vi "Counter.vi"() -> ()   [LabVIEW 2012]
uses:
  <vilib>/DAQmx/read.llb/DAQmx Read (Counter U32 1Chan 1Samp).vi
  <vilib>/DAQmx/create/channels.llb/DAQmx Create Channel (CI-Count Edges).vi
  <vilib>/DAQmx/miscellaneous.llb/DAQmx Fill In Error Info.vi
panel:
  in  "initial count":u32
  out "Det1":u32
  out "Det2":u32
  out "Det3":u32
  out "PSU":u32
  out "error out":errorcluster
  in  "PSU":tag="Dev4/ctr1"
  in  "Det3":tag="Dev4/ctr0"
  in  "Det2":tag="Dev5/ctr1"
  in  "Det1":tag="Dev5/ctr0"
  in  "stop":bool
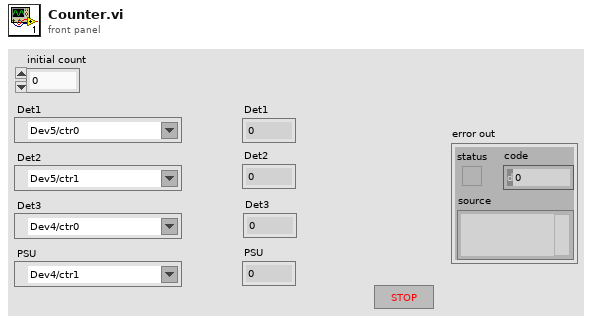
[diagram p1: front panel]
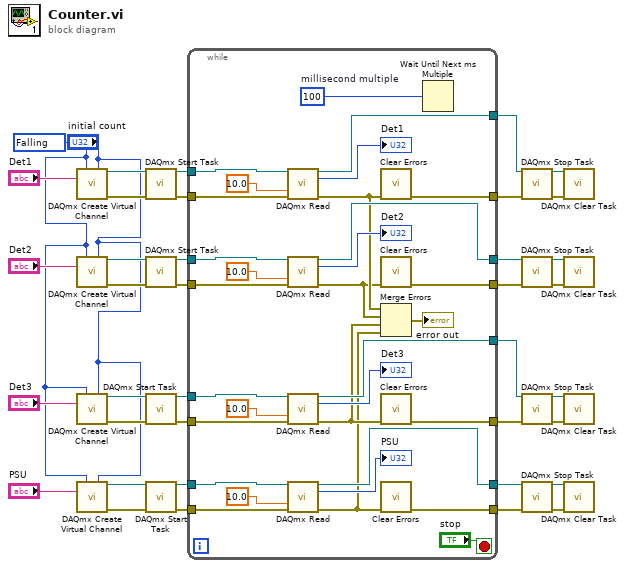
[diagram p0: block diagram]
diagram:
  w1 = 10171 items=["Rising"=10280, "Falling"=10171] ("edge")
  n1 = call-poly <vilib>:"DAQmx Create Virtual Channel.vi"("initial count"="initial count", "edge"=w1, "counter"="Det1") -> ("task out"=w10:refnum<k21>, "error out"=w3:errorcluster)  [unwired: 11 in]
  n2 = call-poly <vilib>:"DAQmx Create Virtual Channel.vi"("initial count"="initial count", "edge"=w1, "counter"="Det2") -> ("task out"=w9:refnum<k21>, "error out"=w4:errorcluster)  [unwired: 11 in]
  n3 = call-poly <vilib>:"DAQmx Create Virtual Channel.vi"("initial count"="initial count", "edge"=w1, "counter"="Det3") -> ("task out"=w8:refnum<k21>, "error out"=w7:errorcluster)  [unwired: 11 in]
  n4 = call-poly <vilib>:"DAQmx Create Virtual Channel.vi"("initial count"="initial count", "edge"=w1, "counter"="PSU") -> ("task out"=w6:refnum<k21>, "error out"=w5:errorcluster)  [unwired: 11 in]
  n5 = call <vilib>:"DAQmx Start Task.vi"("task/channels in"=w10, "error in"=w3) -> ("task out"=w34:refnum<k21>, "error out"=w27:errorcluster)  [unwired: 12 in]
  n6 = call <vilib>:"DAQmx Start Task.vi"("task/channels in"=w9, "error in"=w4) -> ("task out"=w33:refnum<k21>, "error out"=w28:errorcluster)  [unwired: 12 in]
  n7 = call <vilib>:"DAQmx Start Task.vi"("task/channels in"=w8, "error in"=w7) -> ("task out"=w32:refnum<k21>, "error out"=w29:errorcluster)  [unwired: 12 in]
  n8 = call <vilib>:"DAQmx Start Task.vi"("task/channels in"=w6, "error in"=w5) -> ("task out"=w31:refnum<k21>, "error out"=w30:errorcluster)  [unwired: 12 in]
  n9 = while {
    tunnel: w34 -> [w69]
    tunnel: w33 -> [w62]
    tunnel: w32 -> [w60]
    tunnel: w31 -> [w58]
    tunnel: w30 -> [w57]
    tunnel: w29 -> [w59]
    tunnel: w28 -> [w61]
    tunnel: w27 -> [w68]
    tunnel: [w67] -> w26
    tunnel: [w49] -> w25
    tunnel: [w52] -> w24
    tunnel: [w48] -> w23
    tunnel: [w47] -> w21
    tunnel: [w51] -> w22
    tunnel: [w50] -> w20
    tunnel: [w46] -> w19
    stop <- "stop" stop-if-true
    w45 = u32 100  # millisecond multiple
    n10 = call-poly <vilib>:"DAQmx Read.vi"("task/channels in"=w69, "timeout"=10.0, "error in"=w68) -> ("task out"=w67:refnum<k21>, "data"=→"Det1":u32, "error out"=w43:errorcluster)  [unwired: 10 in]
    n11 = call-poly <vilib>:"DAQmx Read.vi"("task/channels in"=w62, "timeout"=10.0, "error in"=w61) -> ("task out"=w52:refnum<k21>, "data"=→"Det2":u32, "error out"=w42:errorcluster)  [unwired: 10 in]
    n12 = call-poly <vilib>:"DAQmx Read.vi"("task/channels in"=w60, "timeout"=10.0, "error in"=w59) -> ("task out"=w51:refnum<k21>, "data"=→"Det3":u32, "error out"=w41:errorcluster)  [unwired: 10 in]
    n13 = call-poly <vilib>:"DAQmx Read.vi"("task/channels in"=w58, "timeout"=10.0, "error in"=w57) -> ("task out"=w50:refnum<k21>, "data"=→"PSU":u32, "error out"=w40:errorcluster)  [unwired: 10 in]
    n14 = call <vilib>:"Clear Errors.vi"("error in (no error)"=w43) -> ("error out"=w49:errorcluster)  [unwired: 6 in]
    n15 = call <vilib>:"Clear Errors.vi"("error in (no error)"=w42) -> ("error out"=w48:errorcluster)  [unwired: 6 in]
    n16 = Merge Errors(w43, w42, w41, w40) -> (→"error out":errorcluster)
    n17 = call <vilib>:"Clear Errors.vi"("error in (no error)"=w41) -> ("error out"=w47:errorcluster)  [unwired: 6 in]
    n18 = call <vilib>:"Clear Errors.vi"("error in (no error)"=w40) -> ("error out"=w46:errorcluster)  [unwired: 6 in]
    n19 = Wait Until Next ms Multiple(millisecond multiple=w45) -> ()  [unwired: 1 out]
  }
  n20 = call <vilib>:"DAQmx Stop Task.vi"("task/channels in"=w26, "error in"=w25) -> ("task out"=w18:refnum<k21>, "error out"=w17:errorcluster)  [unwired: 12 in]
  n21 = call <vilib>:"DAQmx Stop Task.vi"("task/channels in"=w24, "error in"=w23) -> ("task out"=w16:refnum<k21>, "error out"=w15:errorcluster)  [unwired: 12 in]
  n22 = call <vilib>:"DAQmx Stop Task.vi"("task/channels in"=w22, "error in"=w21) -> ("task out"=w14:refnum<k21>, "error out"=w13:errorcluster)  [unwired: 12 in]
  n23 = call <vilib>:"DAQmx Stop Task.vi"("task/channels in"=w20, "error in"=w19) -> ("task out"=w12:refnum<k21>, "error out"=w11:errorcluster)  [unwired: 12 in]
  n24 = call <vilib>:"DAQmx Clear Task.vi"("task in"=w18, "error in"=w17) -> ()  [unwired: 13 in, 1 out]
  n25 = call <vilib>:"DAQmx Clear Task.vi"("task in"=w16, "error in"=w15) -> ()  [unwired: 13 in, 1 out]
  n26 = call <vilib>:"DAQmx Clear Task.vi"("task in"=w14, "error in"=w13) -> ()  [unwired: 13 in, 1 out]
  n27 = call <vilib>:"DAQmx Clear Task.vi"("task in"=w12, "error in"=w11) -> ()  [unwired: 13 in, 1 out]
